vi "Handle New Record.vi"(8 "error in (no error)":errorcluster, 10 "New Record":refnum<class "Record.lvclass">, 11 "Handler in":refnum<class "Handler.lvclass">) -> (0 "error out":errorcluster, 3 "Handler out":refnum<class "Handler.lvclass">)   [LabVIEW 2017, in "Error Log.lvlib" / "Handler.lvclass"]
uses:
  Handler.lvclass
  Record/Record.lvclass
  Record/Record.lvclass/Record.ctl
  Handler.lvclass/Handler.ctl
  Record/Get Level.vi
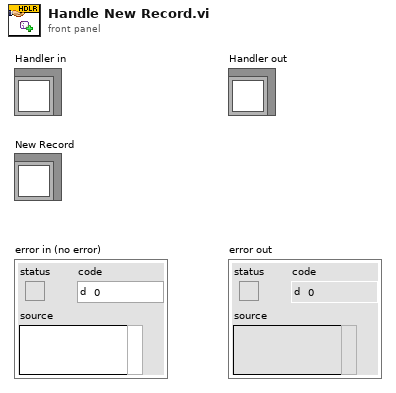
[diagram p1: front panel]
types:
  T1 = enum16{"DEBUG", "INFO", "WARNING", "ERROR", "CRITICAL"}
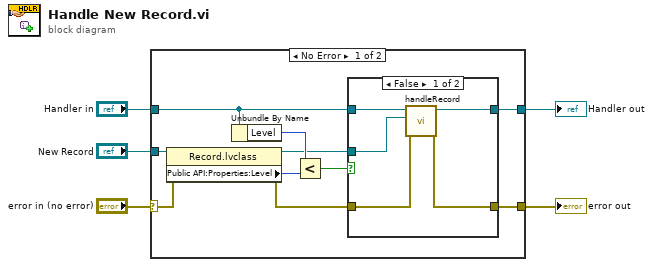
[diagram p0: block diagram]
diagram:
  n1 = case shown="No Error" "error in (no error)" {
    selector: "error in (no error)" -> [w7 w23]
    tunnel: [w15 w23] -> w5
    tunnel: [w14 w24] -> w4
    tunnel: "New Record" -> [w11 _]
    tunnel: "Handler in" -> [w9 w24]
    frame No Error {
      n2 = property class="Record.lvclass"(reference=w11, error in=w7) -> (reference out=w10:refnum<class "Record.lvclass">, error out=w6:errorcluster, "Public API:Properties:Level"=w12:T1)
      n3 = Unbundle By Name(w9) -> ("Level"=w13:T1)
      n4 = Less?(x=w13, y=w12) -> (x < y?=w8:bool)
      n5 = case shown="False" w8 {
        tunnel: [w17 w22] -> w15
        tunnel: [w19 w21] -> w14
        tunnel: w9 -> [w20 w21]
        tunnel: w10 -> [w16 _]
        tunnel: w6 -> [w18 w22]
        frame False {
          n6 = call-dynamic "handleRecord.vi"("error in (no error)"=w18, "Record"=w16, "Handler in"=w20) -> ("error out"=w17:errorcluster, "Handler out"=w19:refnum<class "Handler.lvclass">)  [unwired: 7 in]
        }
        frame True {
        }
      }
    }
    frame Error {
    }
  }
  "error out" <- w5
  "Handler out" <- w4
